vi "PlotCubeParams.vi"() -> ()   [LabVIEW 2014]
uses:
  TypeDefs/RectHatch.ctl
  TypeDefs/PowerSpeed.ctl
  <vilib>/Utility/file.llb/Read From Spreadsheet File (DBL).vi
panel:
  out "OH":T1(array[cluster])=[{-30.0, 30.0, 382.0, 300.0, 114.6, 229.2, 229.2, 382.0, 382.0}, {-15.0, 30.0, 382.0, 300.0, 95.5, 191.0, 286.5, 382.0, 382.0}, {0.0, 30.0, 327.0, 150.0, 98.1, 196.2, 196.2, 327.0, 327.0}, {15.0, 30.0, 382.0, 300.0, 114.6, 229.2, 229.2, 382.0, 382.0}, {30.0, 30.0, 382.0, 300.0, 152.8, 191.0, 229.2, 267.4, 382.0}, {-30.0, 15.0, 382.0, 300.0, 95.5, 191.0, 286.5, 382.0, 382.0}, {-15.0, 15.0, 327.0, 150.0, 81.75, 163.5, 245.25, 327.0, 327.0}, {0.0, 15.0, 382.0, 300.0, 152.8, 191.0, 229.2, 267.4, 382.0}, {15.0, 15.0, 327.0, 150.0, 130.8, 163.5, 196.2, 228.9, 327.0}, {30.0, 15.0, 382.0, 300.0, 114.6, 229.2, 229.2, 382.0, 382.0}, {-30.0, 0.0, 327.0, 150.0, 98.1, 196.2, 196.2, 327.0, 327.0}, {-15.0, 0.0, 382.0, 300.0, 95.5, 191.0, 286.5, 382.0, 382.0}, {0.0, 0.0, 327.0, 150.0, 81.75, 163.5, 245.25, 327.0, 327.0}, {15.0, 0.0, 382.0, 300.0, 152.8, 191.0, 229.2, 267.4, 382.0}, {30.0, 0.0, 327.0, 150.0, 130.8, 163.5, 196.2, 228.9, 327.0}, {-30.0, -15.0, 382.0, 300.0, 114.6, 229.2, 229.2, 382.0, 382.0}, {-15.0, -15.0, 327.0, 150.0, 98.1, 196.2, 196.2, 327.0, 327.0}, {0.0, -15.0, 382.0, 300.0, 95.5, 191.0, 286.5, 382.0, 382.0}, {15.0, -15.0, 327.0, 150.0, 81.75, 163.5, 245.25, 327.0, 327.0}, {30.0, -15.0, 382.0, 300.0, 152.8, 191.0, 229.2, 267.4, 382.0}, {-30.0, -30.0, 382.0, 300.0, 114.6, 229.2, 229.2, 382.0, 382.0}, {-15.0, -30.0, 382.0, 300.0, 95.5, 191.0, 286.5, 382.0, 382.0}, {0.0, -30.0, 327.0, 150.0, 130.8, 163.5, 196.2, 228.9, 327.0}, {15.0, -30.0, 382.0, 300.0, 152.8, 191.0, 229.2, 267.4, 382.0}, {30.0, -30.0, 327.0, 150.0, 98.1, 196.2, 196.2, 327.0, 327.0}]
  in  "DummyCubeLoc":cluster{dbl, dbl}={-45.0, 30.0}
  in  "Save?":bool
  in  "Path":path=path "\\\\nif-prgms-srvr.llnl.gov\\LMOT/Damage Group/Matthews/AM/fraunhofer SLM/BuildFiles_STL_ILT/SCN/OHparam_11-18-16"
  in  "HighPower":dbl=500.0
  in  "Display":T2={"Mode"=enum."Inherit Value", "PointSize"=1.0, "LineWidth"=1.0}
  in  "LayerEnd":u32=170
  in  "LayerStart":u32=170
  in  "HatchPow":T3={"Power"=300.0, "Mark Speed"=400.0, "Jump Speed"=1000.0, "JumpPower"=0.0}
  in  "RectHatch":T4={"Width"=10.0, "Height"=10.0, "Angle"=45.0, "OffX"=0.1, "OffY"=0.1, "Spacing"=0.1, "IslandSize"=0.1} {"IslandSize" format="%#_13g"; "Spacing" format="%#_13g"; "OffY" format="%#_13g"; "OffX" format="%#_13g"; "Height" format="%#_13g"; "Width" format="%#_13g"}
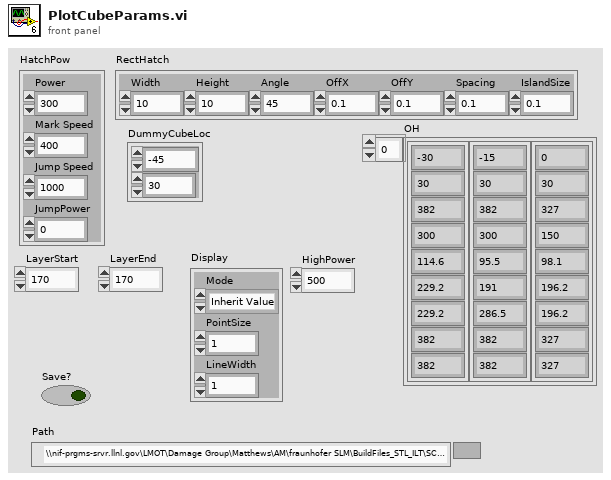
[diagram p1: front panel]
types:
  T1 = cluster{dbl, dbl, dbl, dbl, dbl, dbl, dbl, dbl, dbl}[]
  T2 = cluster{"Mode":enum16{"Inherit Value", "Points", "Wireframe", "Polygons"}, "PointSize":sgl, "LineWidth":sgl}
  T3 = typedef "PowerSpeed.ctl" = cluster{"Power":dbl, "Mark Speed":dbl, "Jump Speed":dbl, "JumpPower":dbl}
  T4 = typedef "RectHatch.ctl" = cluster{"Width":dbl, "Height":dbl, "Angle":sgl, "OffX":dbl, "OffY":dbl, "Spacing":dbl, "IslandSize":dbl}
  T5 = cluster{dbl, dbl, dbl, dbl, dbl, dbl, dbl, dbl, dbl}
  T6 = typedef "PathSupreme.ctl" = cluster{"VelocityProfiles":T7[], "Path":T8}
  T7 = typedef "VelocityProfile.ctl" = cluster{"ID":u32, "Velocity":dbl, "Mode":string, "tV1":u32, "tV2":u32, "tL1":u32, "tL2":u32}
  T8 = typedef "PathCut.ctl" = cluster{"Type":string, "Tag":string, "Segments":T9[]}
  T9 = typedef "Segment.ctl" = cluster{"SegmentID":u16, "Power":sgl, "idxVelocityProfile":u16, "End":cluster{"X":sgl, "Y":sgl}}
  T10 = typedef "Point3D.ctl" = cluster{"X":sgl, "Y":sgl, "Z":sgl}
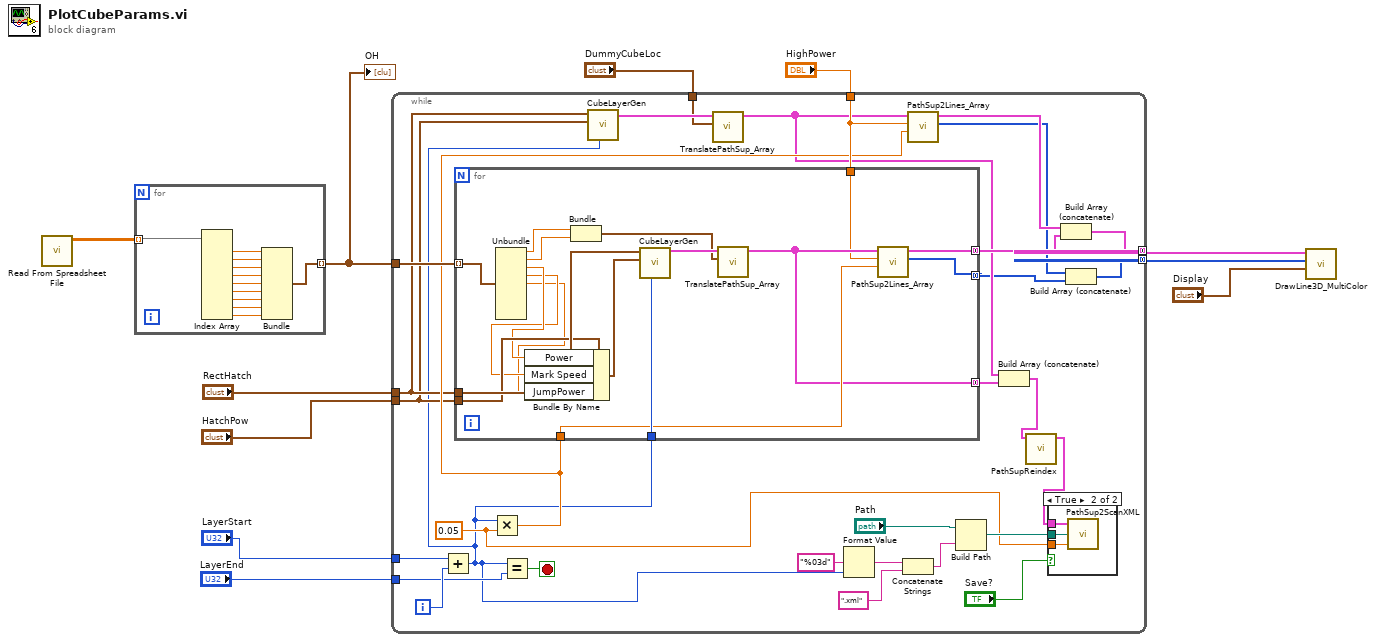
[diagram p0: block diagram]
diagram:
  n1 = call-poly <vilib>:"Read From Spreadsheet File.vi"() -> ("all rows"=w11:dbl[][])  [unwired: 7 in, 4 out]
  n2 = for {
    tunnel: w11 -> [w22] mode=indexing
    tunnel: [w17] -> w6 mode=indexing
    n3 = Index Array(array=w22) -> (element #1=w20:dbl, element #2=w21:dbl, element #3=w19:dbl, element #4=w18:dbl, element #5=w16:dbl, element #6=w15:dbl, element #7=w14:dbl, element #8=w13:dbl, element #9=w12:dbl)  [unwired: 9 in]
    n4 = Bundle(w20, w21, w19, w18, w16, w15, w14, w13, w12) -> (w17:T5)  [unwired: 1 in]
  }
  "OH" <- w6
  n5 = while {
    tunnel: "HighPower" -> [w37]
    tunnel: [w33] -> w9 mode=concatenating
    tunnel: [w32] -> w8 mode=concatenating
    tunnel: w6 -> [w50]
    tunnel: "RectHatch" -> [w29]
    tunnel: "HatchPow" -> [w28]
    tunnel: "LayerEnd" -> [w49]
    tunnel: "LayerStart" -> [w48]
    tunnel: "DummyCubeLoc" -> [w38]
    i -> [w52]
    stop <- w51 stop-if-true
    w41 = 0.05 ("y")
    n6 = Add(x=w48, y=w52) -> (x+y=w27:u32)
    n7 = Multiply(x=w27, y=w41) -> (x*y=w36:dbl)
    n8 = for {
      tunnel: w27 -> [w72]
      tunnel: w36 -> [w66]
      tunnel: w37 -> [w62]
      tunnel: [w71] -> w34 mode=concatenating
      tunnel: w50 -> [w70] mode=indexing
      tunnel: w29 -> [w69]
      tunnel: w28 -> [w60]
      tunnel: [w63] -> w31 mode=concatenating
      tunnel: [w61] -> w26 mode=concatenating
      n9 = Unbundle(w70) -> (w68:dbl, w67:dbl, w58:dbl, w57:dbl, w56:dbl)  [unwired: 4 out]
      n10 = Bundle By Name(cluster=w60, "Power"=w58, "Mark Speed"=w57, "JumpPower"=w56) -> (w59:T3)
      n11 = Bundle(w68, w67) -> (w64:cluster{dbl, dbl})  [unwired: 1 in]
      n12 = call "CubeLayerGen.vi"("Layer"=w72, "HatchPow"=w59, "RectHatch"=w69) -> ("PathSups"=w65:T6[])  [unwired: 8 in]
      n13 = call "TranslatePathSup_Array.vi"("Offset"=w64, "PathSupsIn"=w65) -> ("PathSupsOut"=w63:T6[])  [unwired: 9 in]
      n14 = call "PathSup2Lines_Array.vi"("Z"=w66, "HighPower"=w62, "PathSupIn"=w63) -> ("Colors"=w61:u32[], "Lines"=w71:cluster{"P0":T10, "P1":T10}[])  [unwired: 7 in]
    }
    n15 = Equal?(x=w27, y=w49) -> (x = y?=w51:bool)
    n16 = call "CubeLayerGen.vi"("Layer"=w27, "HatchPow"=w28, "RectHatch"=w29) -> ("PathSups"=w39:T6[])  [unwired: 8 in]
    n17 = call "TranslatePathSup_Array.vi"("Offset"=w38, "PathSupsIn"=w39) -> ("PathSupsOut"=w30:T6[])  [unwired: 9 in]
    n18 = Format Value(format string="%03d", value (0)=w27) -> (output string=w46:string)  [unwired: 1 in]
    n19 = Concatenate Strings(w46, ".xml" ("string")) -> (w44:string)
    n20 = call "PathSup2Lines_Array.vi"("Z"=w36, "HighPower"=w37, "PathSupIn"=w30) -> ("Colors"=w25:u32[], "Lines"=w35:cluster{"P0":T10, "P1":T10}[])  [unwired: 7 in]
    n21 = Build Path(base path="Path", name or relative path=w44) -> (appended path=w42:path)
    n22 = Build Array (concatenate)(w30, w31) -> (w24:T6[])
    n23 = call "PathSupReindex.vi"("PathSupremes"=w24) -> ("PathSupOut"=w23:T6[])  [unwired: 10 in]
    n24 = case shown="True" "Save?" {
      tunnel: w23 -> [_ w55]
      tunnel: w42 -> [_ w54]
      tunnel: w41 -> [_ w53]
      frame False {
      }
      frame True {
        n25 = call "PathSup2ScanXML.vi"("Thickness"=w53, "Path"=w54, "PathSupremes"=w55) -> ()  [unwired: 2 in, 1 out]
      }
    }
    n26 = Build Array (concatenate)(w35, w34) -> (w33:cluster{"P0":T10, "P1":T10}[])
    n27 = Build Array (concatenate)(w25, w26) -> (w32:u32[])
  }
  n28 = call "DrawLine3D_MultiColor.vi"("Display"="Display", "Colors"=w8, "Lines"=w9) -> ()  [unwired: 9 in]
